vi "SetAutoControlActive.vi"(2 "AutoControlActive":bool) -> ()   [LabVIEW 2017]
uses:
  <vilib>/Rock Robotics/Network Tables/NT Write Boolean.vi
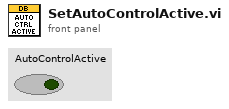
[diagram p1: front panel]
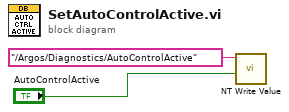
[diagram p0: block diagram]
diagram:
  n1 = call-poly <vilib>:"NT Write Value.vi"("Boolean"="AutoControlActive", "Name"="/Argos/Diagnostics/AutoControlActive") -> ()  [unwired: 9 in, 1 out]
